vi "Measurement UI.vi"() -> ()   [LabVIEW 2021, in "Eff And Load Reg_Channel Ganging_UI.lvlib"]
uses:
  Eff And Load Reg_Channel Ganging_UI.lvlib
panel:
  in  "MeasGraphs":T1(tab)
  out "EfficiencyGraph":T2(graph)
  out "LoadRegulationGraph(V/A)":T3(graph)
  out "LoadRegulationGraph(%)":T3(graph)
  out "Load voltage deviation":dbl[](array[numeric])
  out "Ganged load voltages":dbl[](array[numeric])
  in  "Load current pole-zero ratio":dbl=0.3
  in  "Load current compensation frequency":dbl=180000.0
  in  "Load current gain bandwidth":dbl=14000.0
  in  "Source voltage pole-zero ratio":dbl=2.0
  in  "Source voltage compensation frequency":dbl=3530.0
  in  "Source voltage gain bandwidth":dbl=2000.0
  in  "Load resource names":string[](array[string])
  in  "Source resource names":string[](array[string])
  out "Load sweep points":i32
  out "Source sweep points":i32
  out "Voltage values":dbl[](array[numeric])
  out "Efficiency":dbl[](array[numeric])
  out "Ganged load currents":dbl[](array[numeric])
  in  "Mode of operation":T4(ring)
  in  "ModeOfConfiguration":T5(tab)
  in  "DEVICE POWER":bool=TRUE
  out "Status":string
  in  "Load config power on":string="Load Config"
  in  "POWERON/OFFLOADResourceNames":refnum<k15>[](array[refnum]) caption="RESOURCE NAMES"
  in  "Source config power on":string="Source Config"
  in  "POWERON/ OFFSOURCEResourceNames":refnum<k15>[](array[refnum]) caption="RESOURCE NAMES\n(Single/Master & Slave)"
  in  "Power on source sense":i32(ring)=1009 caption="SENSE" items=["Local"=1008, "Remote"=1009]
  in  "Power on/off Source voltage/current limit range":dbl=15.0 caption="CURRENT LIMIT" format="%#_6pA"
  in  "Power on/off Source voltage/current level":dbl=6.0 caption="VOLTAGE LEVEL" format="%#_6pV"
  in  "Power on source system configuration":enum32{"Series", "Parallel"}(ring)=enum."Parallel" caption="SYSTEM CONFIG"
  in  "Power ON output function":i32(ring)=1006 caption="OUTPUT FUNCTION" items=["DC Voltage"=1006, "DC Current"=1007]
  in  "MeasConfigurations":T6(tab)=enum."Source Config"
  in  "Measurement timeout":dbl=10.0 caption="MEASUREMENT TIME-OUT" format="%.3ps"
  in  "Nominal output voltage":dbl=1.0 caption="NOMINAL OUTPUT VOLTAGE" format="%.3fV"
  in  "Source delay":dbl=0.005 caption="SOURCE DELAY" format="%.3ps"
  in  "DUT setup time":dbl=1.0 caption="DUT SETUP TIME" format="%.3ps"
  in  "Aperture time":dbl=0.005 caption="APERTURE TIME" format="%.3ps"
  in  "PPSSResourceNames":refnum<k15>[](array[refnum]) caption="RESOURCE NAMES"
  in  "Source stop voltage":dbl=14.0 caption="VOLTAGE STOP LEVEL" format="%#_6pV"
  in  "Source transient response":i32(ring)=1038 caption="TRANSIENT RESPONSE" items=["Slow"=1041, "Normal"=1038, "Fast"=1039, "Custom"=1042]
  in  "Power ON/Source sense":i32(ring)=1009 caption="SENSE" items=["Local"=1008, "Remote"=1009]
  in  "Source voltage level range":dbl=20.0 caption="VOLTAGE LEVEL RANGE" format="%#_6pV"
  in  "Power ON V/I Source start level":dbl=6.0 caption="VOLTAGE START LEVEL" format="%#_6pV"
  in  "Source current limit high":dbl=25.0 caption="CURRENT LIMIT/LIMIT HIGH" format="%#_6pA"
  in  "Power ON/Source current/voltage limit range":dbl=25.0 caption="CURRENT LIMIT RANGE" format="%#_6pA"
  in  "Source limit symmetry":enum32{"Symmetric", "Asymmetric"}(ring)=enum."Asymmetric" caption="LIMIT SYMMETRY"
  in  "Source current limit low":dbl=-0.6 caption="CURRENT LIMIT LOW" format="%#_6pA"
  in  "Power ON/Source system configuration":enum32{"Series", "Parallel"}(ring)=enum."Parallel" caption="SYSTEM CONFIG"
  in  "Source compliance":string="Compliance"
  in  "Source sourceadapt":string="SourceAdapt"
  in  "Source voltage sweep points":i32=4 caption="NO. OF POINTS"
  in  "Source Custom Transient Response":bool
  in  "Load current sweep points/points per decade":i32=10 caption="PTS/PTS PER DECADE"
  in  "Load sweep type":string(combo)="Logarithmic" caption="SWEEP TYPE"
  in  "Load stop current":dbl=50.0 caption="CURRENT STOP LEVEL" format="%#_6pA"
  in  "Load sourceadapt":string="SourceAdapt"
  in  "Load compliance":string="Compliance"
  in  "Load system configuration":enum32{"Series", "Parallel"}(ring)=enum."Parallel" caption="SYSTEM CONFIG"
  in  "Load voltage limit low":dbl caption="VOLTAGE  LIMIT LOW" format="%#_6pV"
  in  "Load limit symmetry":enum32{"Symmetric", "Asymmetric"}(ring) caption="LIMIT SYMMETRY"
  in  "Load voltage limit range":dbl=6.0 caption="VOLTAGE LIMIT RANGE" format="%#_6pV"
  in  "Load voltage limit high":dbl=inf caption="VOLTAGE LIMIT/LIMIT HIGH" format="%#_6p"
  in  "Load start current":dbl=2.0 caption="CURRENT START LEVEL" format="%#_6pA"
  in  "Load current level range":dbl=80.0 caption="CURRENT LEVEL RANGE" format="%#_6pA"
  in  "Load sense":i32(ring)=1009 caption="SENSE" items=["Local"=1008, "Remote"=1009]
  in  "Load transient response":i32(ring)=1038 caption="TRANSIENT RESPONSE" items=["Slow"=1041, "Normal"=1038, "Fast"=1039, "Custom"=1042]
  in  "ELoad resource names":refnum<k15>[](array[refnum]) caption="RESOURCE NAMES"
  in  "Load Custom Transient Response":bool
  in  "Load device voltage/current rating":dbl=50.0 caption="DEVICE CURRENT RATING" format="%#_6pA"
  out "Eload status":string
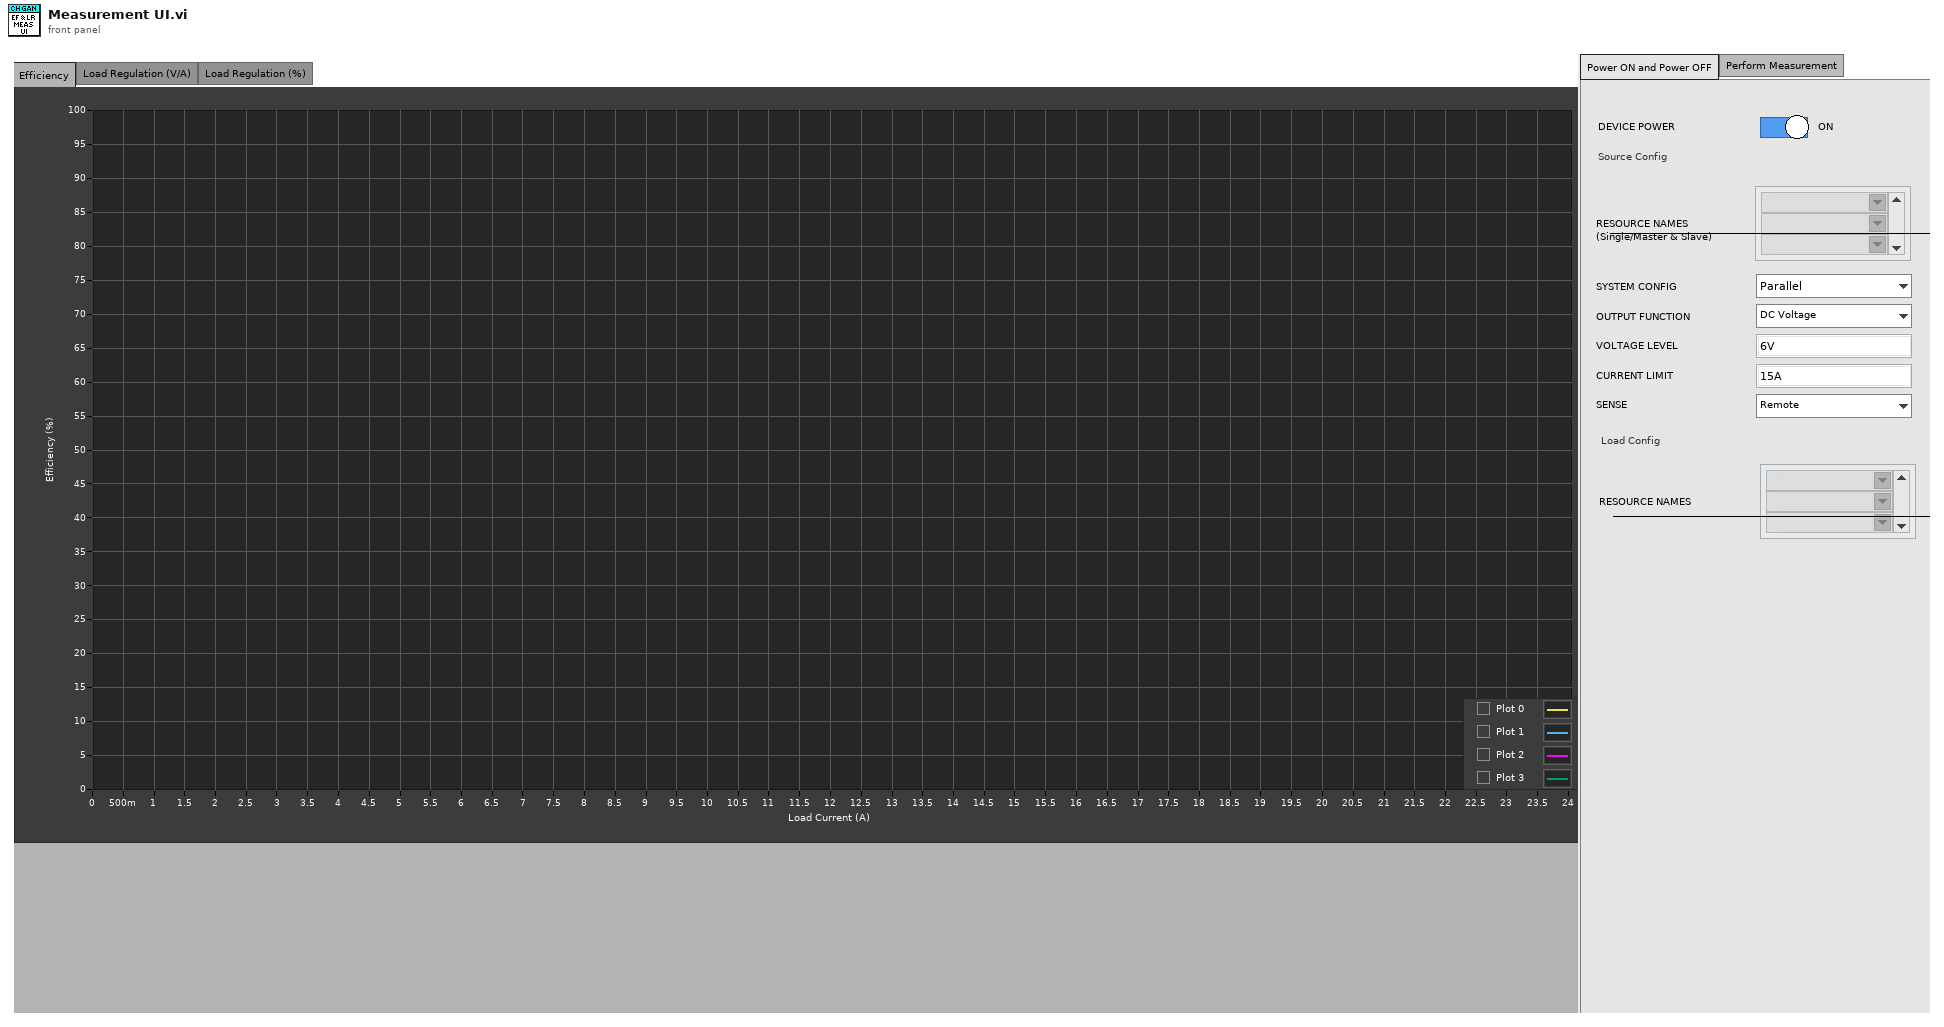
[diagram p1: front panel]
types:
  T1 = enum32{"Efficiency", "Load Regulation (V/A)", "Load Regulation (%)", "Hidden Controls"}
  T2 = cluster{"Ganged load currents":dbl[], "Efficiency":dbl[]}[]
  T3 = cluster{"Load currents":dbl[], "Efficiency":dbl[]}[]
  T4 = enum32{"Power on the DUT", "Perform measurement", "Power off the DUT"}
  T5 = enum32{"Power ON and Power OFF", "Perform Measurement"}
  T6 = enum32{"Measurement Config", "Source Config", "Load Config"}
  T7 = typedef "SourceAdapt Parameters.ctl" = cluster{"Voltage gain bandwidth":dbl, "Voltage compensation frequency":dbl, "Voltage pole-zero ratio":dbl, "Current gain bandwidth":dbl, "Current compensation frequency":dbl, "Current pole-zero ratio":dbl}
  T8 = cluster{"Ganged load currents":dbl[], "Efficiency":dbl[]}
  T9 = cluster{"Ganged load currents":dbl[], "Ganged load voltages":dbl[]}
  T10 = cluster{"Ganged load currents":dbl[], "Load voltage deviation":dbl[]}
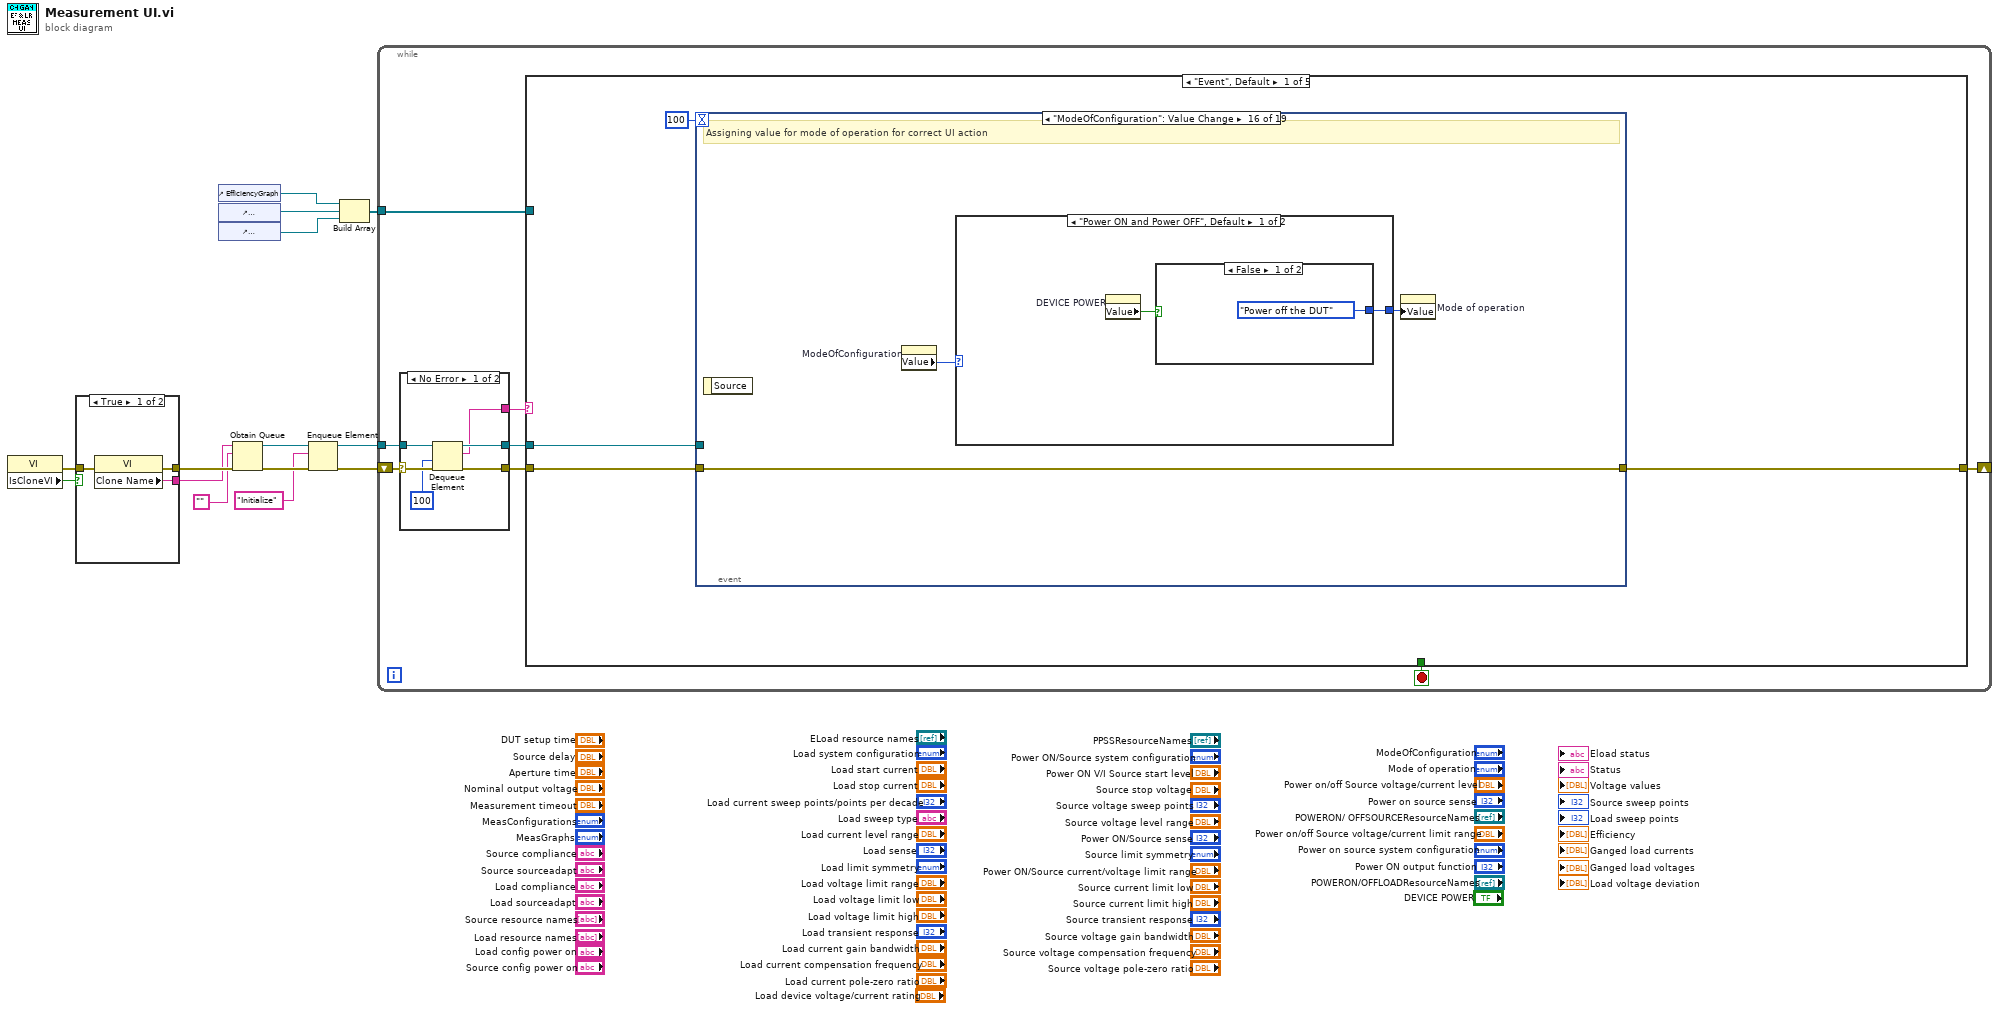
[diagram p0: block diagram]
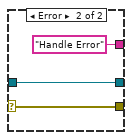
[diagram p2: hidden frame]
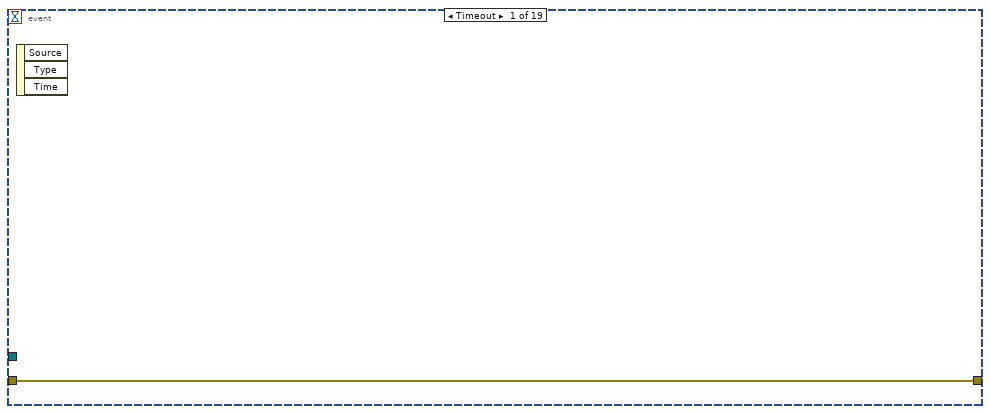
[diagram p3: hidden frame]
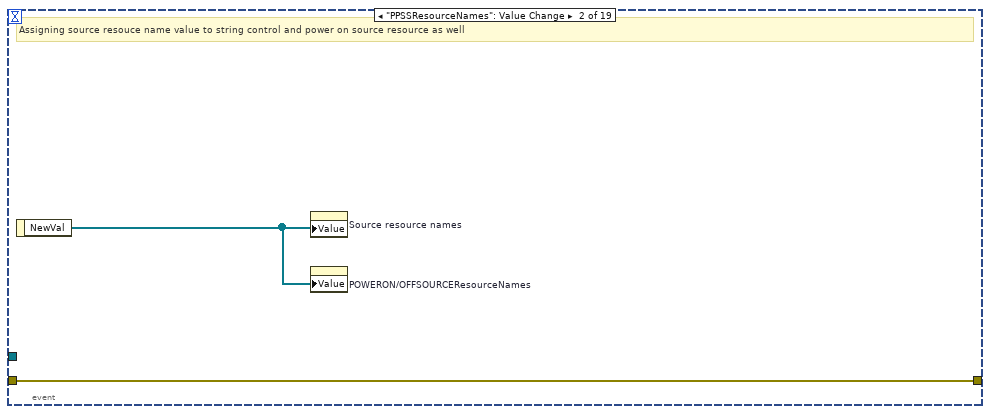
[diagram p4: hidden frame]
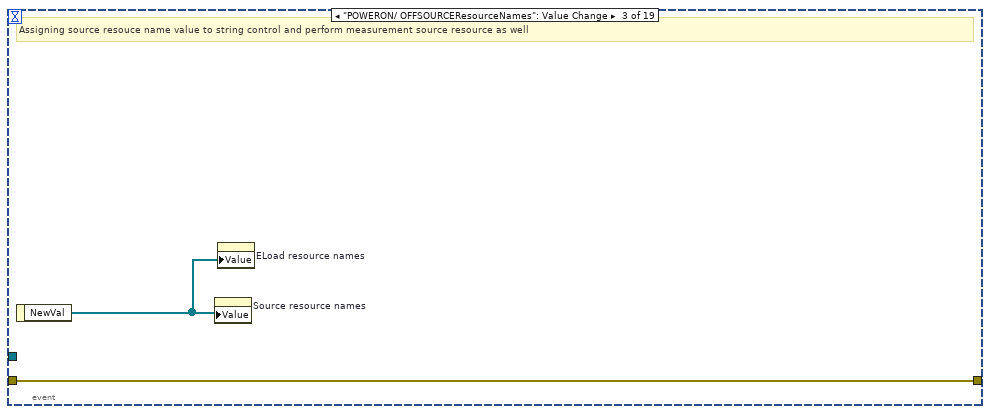
[diagram p5: hidden frame]
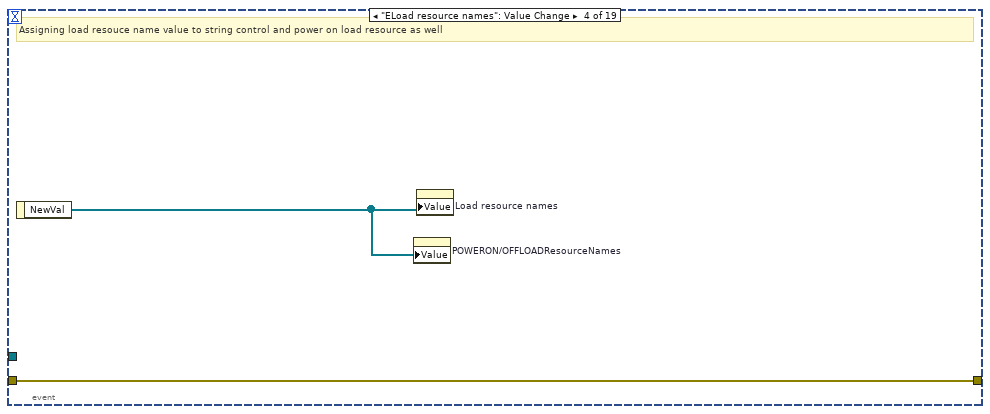
[diagram p6: hidden frame]
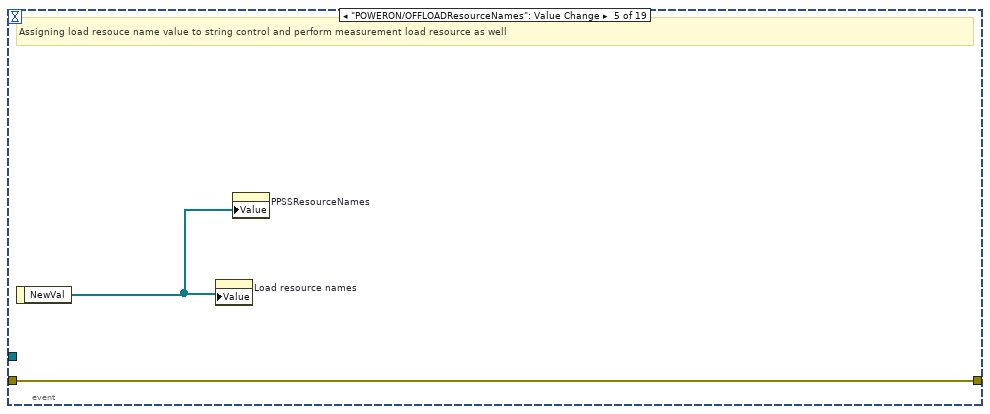
[diagram p7: hidden frame]
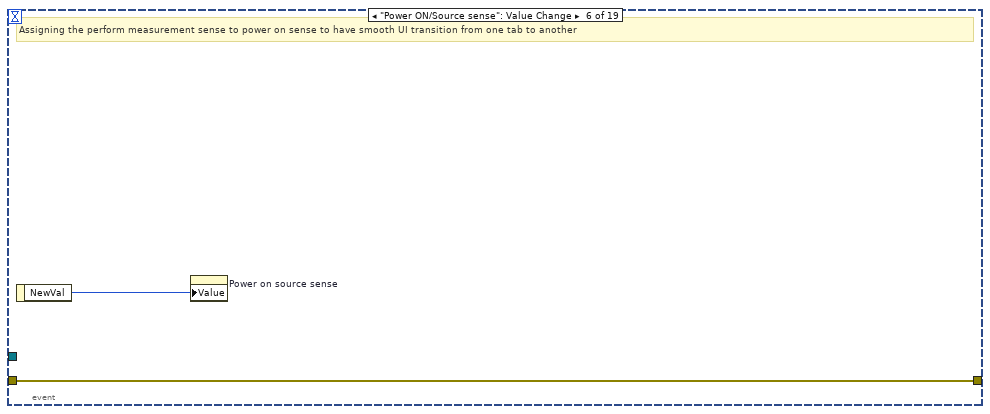
[diagram p8: hidden frame]
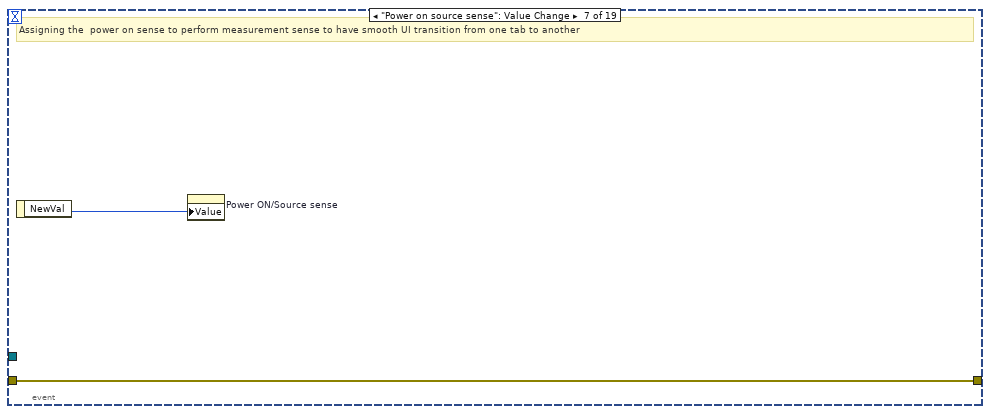
[diagram p9: hidden frame]
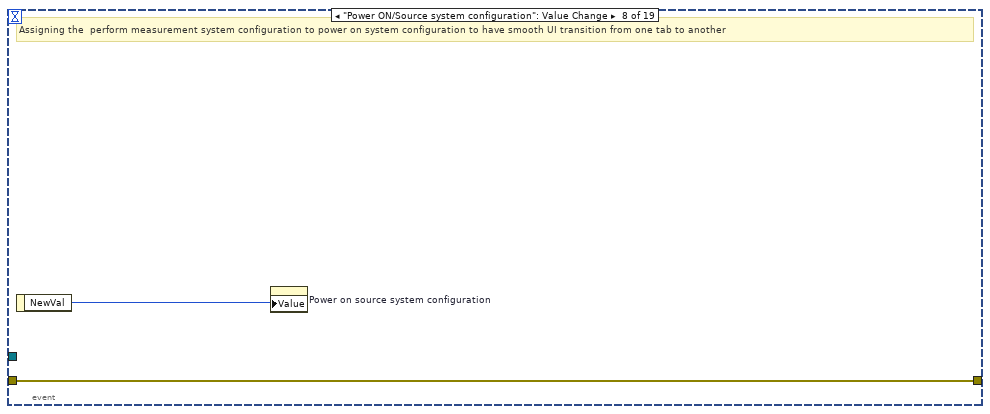
[diagram p10: hidden frame]
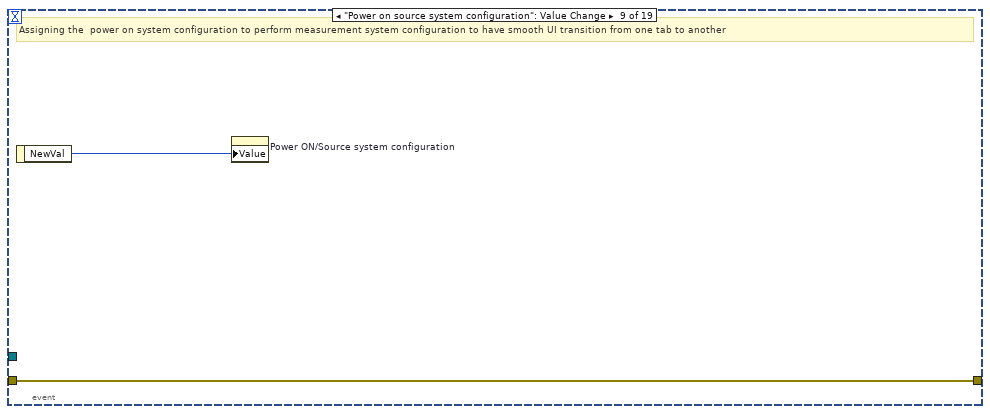
[diagram p11: hidden frame]
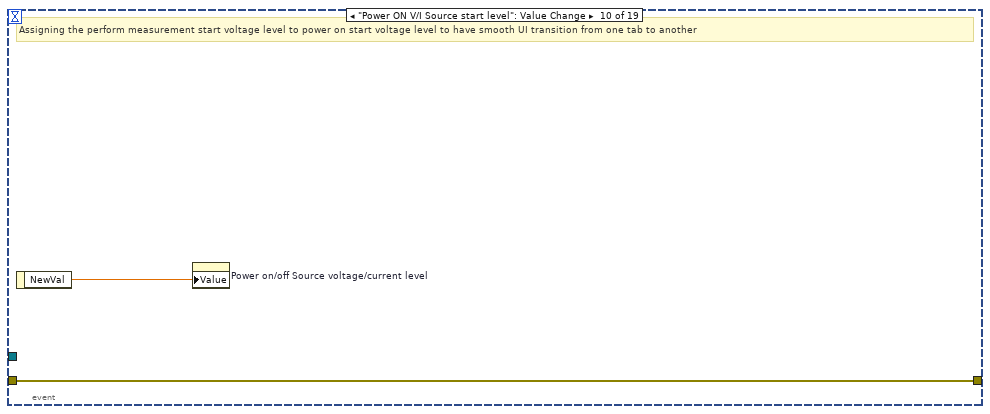
[diagram p12: hidden frame]
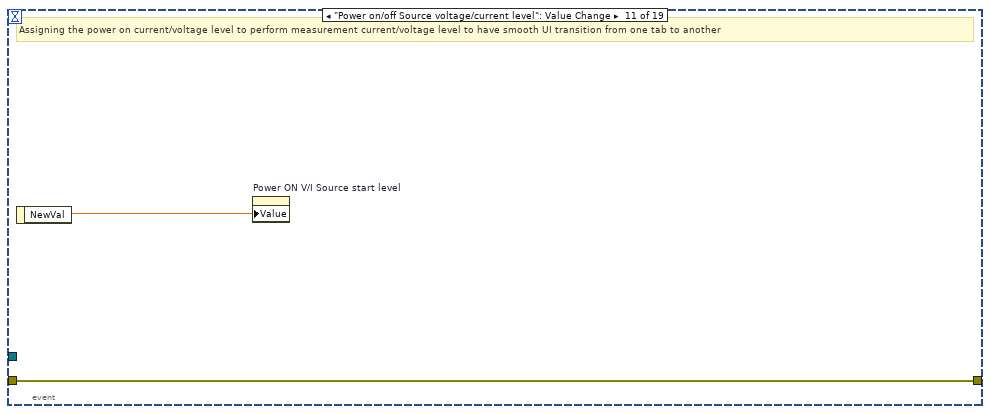
[diagram p13: hidden frame]
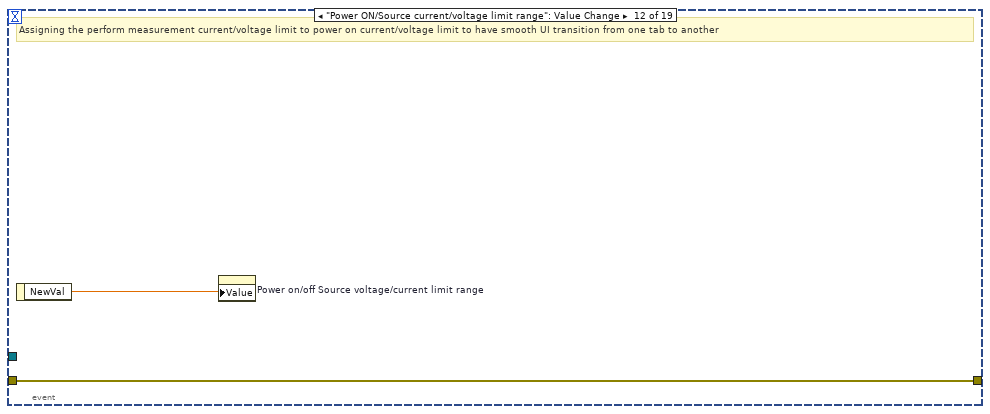
[diagram p14: hidden frame]
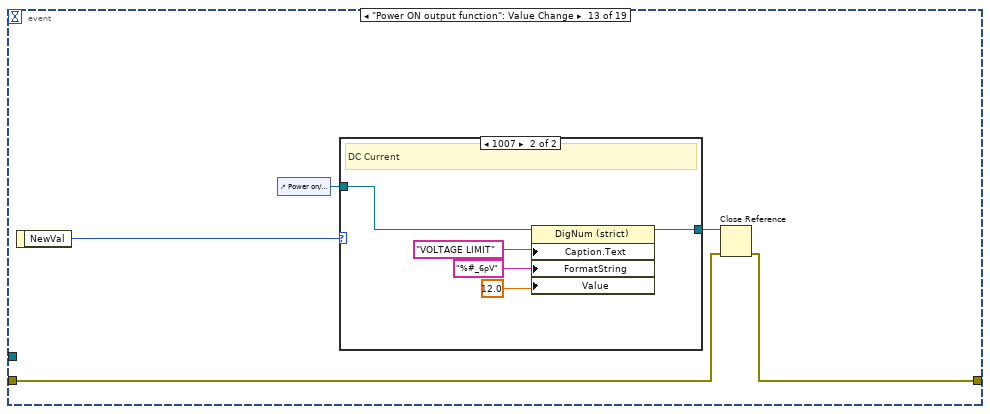
[diagram p15: hidden frame]
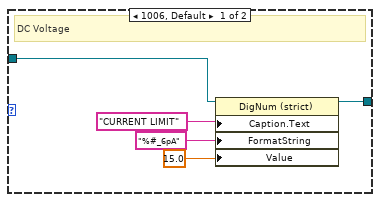
[diagram p16: hidden frame]
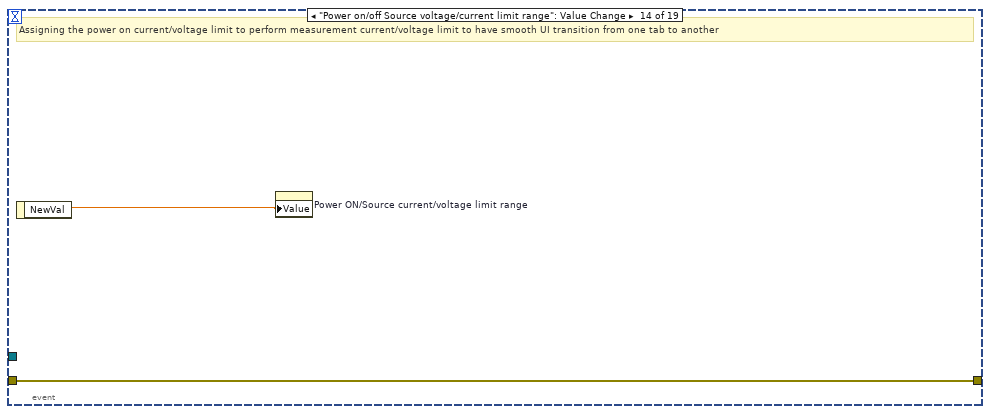
[diagram p17: hidden frame]
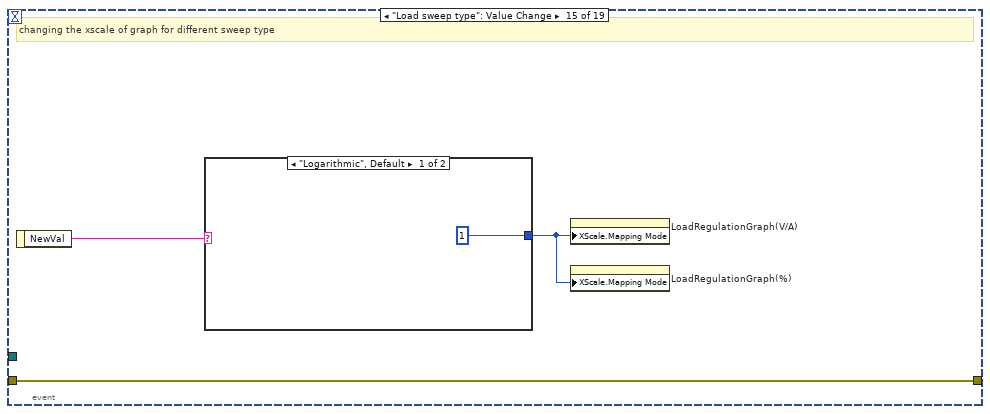
[diagram p18: hidden frame]
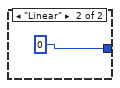
[diagram p19: hidden frame]
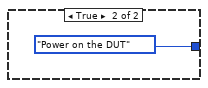
[diagram p20: hidden frame]
diagram:
  n1 = property class="VI"() -> (error out=w5:errorcluster, "IsCloneVI"=w6:bool)  [unwired: 2 in, 1 out]
  n2 = case shown="True" w6 {
    tunnel: [w17 w20] -> w14
    tunnel: [w16 w19] -> w13
    tunnel: w5 -> [w15 w18]
    frame True {
      n3 = property class="VI"(error in=w15) -> (error out=w17:errorcluster, "Clone Name"=w16:string)  [unwired: 1 in, 1 out]
    }
    frame False {
      n4 = property class="VI"(error in=w18) -> (error out=w20:errorcluster, "Name"=w19:string)  [unwired: 1 in, 1 out]
    }
  }
  n5 = control-ref of="EfficiencyGraph"() -> (w2:refnum<vi>)
  n6 = control-ref of="LoadRegulationGraph(V/A)"() -> (w3:refnum<vi>)
  n7 = control-ref of="LoadRegulationGraph(%)"() -> (w4:refnum<vi>)
  n8 = Obtain Queue(name (unnamed)=w13, element data type="", error in (no error)=w14) -> (queue out=w10:refnum<queue>, error out=w12:errorcluster)  [unwired: 2 in, 1 out]
  n9 = Enqueue Element(queue=w10, element="Initialize", error in (no error)=w12) -> (queue out=w9:refnum<queue>, error out=w11:errorcluster)  [unwired: 1 in, 1 out]
  n10 = Build Array(w2, w3, w4) -> (w1:refnum<vi>[])
  n11 = while {
    shift-right: [w23] -> _
    shift-left: w11 -> [w28]
    tunnel: w9 -> [w26]
    tunnel: w1 -> [w21]
    stop <- w22 stop-if-true
    n12 = case shown="No Error" w28 {
      selector: w28 -> [w34 w37]
      tunnel: [w33 w37] -> w27
      tunnel: w26 -> [w32 w36]
      tunnel: [w31 w36] -> w25
      tunnel: [w30 "Handle Error"] -> w24
      frame No Error {
        n13 = Dequeue Element(queue=w32, timeout in ms (-1)=100, error in (no error)=w34) -> (queue out=w31:refnum<queue>, element=w30:string, error out=w33:errorcluster)  [unwired: 1 out]
      }
      frame Error {
      }
    }
    n14 = case shown="\"Event\", Default" w24 {
      tunnel: w27 -> [w40 w110 w125 w182 w183]
      tunnel: w25 -> [w38 _ _ w180 _]
      tunnel: [w41 w110 w125 w177 w183] -> w23
      tunnel: [_ _ _ TRUE _] -> w22
      tunnel: w21 -> [_ _ w113 _ _]
      frame "Event", Default {
        n15 = event shown="[15] \"ModeOfConfiguration\": Value Change" {
          selector: _ -> [_ _ _ _ _ _ _ _ _ _ _ _ _ _ _ _ _ _ _]
          dyn-events: _ -> [_ _ _ _ _ _ _ _ _ _ _ _ _ _ _ _ _ _ _]
          timeout: 100 -> [_ _ _ _ _ _ _ _ _ _ _ _ _ _ _ _ _ _ _]
          tunnel: [w42 w44 w46 w48 w49 w51 w53 w55 w57 w59 w61 w63 w65 w81 w82 w87 w98 w103 w107] -> w41
          tunnel: w40 -> [w42 w44 w46 w48 w49 w51 w53 w55 w57 w59 w61 w63 w66 w81 w82 w87 w98 w103 w108]
          tunnel: w38 -> [_ _ _ _ _ _ _ _ _ _ _ _ _ _ _ _ _ _ w106]
          event Timeout {
            n16 = event-data() -> ()  [unwired: 1 in, 3 out]
          }
          event "PPSSResourceNames": Value Change {
            # "Assigning source resouce name value to string control and power on source resource as well"
            n17 = event-data() -> ("NewVal"=w43:refnum<k15>[])  [unwired: 1 in]
            n18 = property on="Source resource names" class="Arr (strict)"("Value"=w43) -> ()  [unwired: 2 in, 2 out]
            n19 = property on="POWERON/OFFSOURCEResourceNames" class="Arr (strict)"("Value"=w43) -> ()  [unwired: 2 in, 2 out]
          }
          event "POWERON/ OFFSOURCEResourceNames": Value Change {
            # "Assigning source resouce name value to string control and perform measurement source resource as well"
            n20 = event-data() -> ("NewVal"=w45:refnum<k15>[])  [unwired: 1 in]
            n21 = property on="Source resource names" class="Arr (strict)"("Value"=w45) -> ()  [unwired: 2 in, 2 out]
            n22 = property on="ELoad resource names" class="Arr (strict)"("Value"=w45) -> ()  [unwired: 2 in, 2 out]
          }
          event "ELoad resource names": Value Change {
            # "Assigning load resouce name value to string control and power on load resource as well"
            n23 = event-data() -> ("NewVal"=w47:refnum<k15>[])  [unwired: 1 in]
            n24 = property on="POWERON/OFFLOADResourceNames" class="Arr (strict)"("Value"=w47) -> ()  [unwired: 2 in, 2 out]
            n25 = property on="Load resource names" class="Arr (strict)"("Value"=w47) -> ()  [unwired: 2 in, 2 out]
          }
          event "POWERON/OFFLOADResourceNames": Value Change {
            # "Assigning load resouce name value to string control and perform measurement load resource as well"
            n26 = event-data() -> ("NewVal"=w50:refnum<k15>[])  [unwired: 1 in]
            n27 = property on="Load resource names" class="Arr (strict)"("Value"=w50) -> ()  [unwired: 2 in, 2 out]
            n28 = property on="PPSSResourceNames" class="Arr (strict)"("Value"=w50) -> ()  [unwired: 2 in, 2 out]
          }
          event "Power ON/Source sense": Value Change {
            # "Assigning the perform measurement sense to power on sense to have smooth UI transition from one tab to another"
            n29 = event-data() -> ("NewVal"=w52:i32)  [unwired: 1 in]
            n30 = property on="Power on source sense" class="Ring (strict)"("Value"=w52) -> ()  [unwired: 2 in, 2 out]
          }
          event "Power on source sense": Value Change {
            # "Assigning the  power on sense to perform measurement sense to have smooth UI transition from one tab to another"
            n31 = event-data() -> ("NewVal"=w54:i32)  [unwired: 1 in]
            n32 = property on="Power ON/Source sense" class="Ring (strict)"("Value"=w54) -> ()  [unwired: 2 in, 2 out]
          }
          event "Power ON/Source system configuration": Value Change {
            # "Assigning the  perform measurement system configuration to power on system configuration to have smooth UI transition from one tab to another"
            n33 = event-data() -> ("NewVal"=w56:enum32{"Series", "Parallel"})  [unwired: 1 in]
            n34 = property on="Power on source system configuration" class="Enum (strict)"("Value"=w56) -> ()  [unwired: 2 in, 2 out]
          }
          event "Power on source system configuration": Value Change {
            # "Assigning the  power on system configuration to perform measurement system configuration to have smooth UI transition from one tab to another"
            n35 = event-data() -> ("NewVal"=w58:enum32{"Series", "Parallel"})  [unwired: 1 in]
            n36 = property on="Power ON/Source system configuration" class="Enum (strict)"("Value"=w58) -> ()  [unwired: 2 in, 2 out]
          }
          event "Power ON V/I Source start level": Value Change {
            # "Assigning the perform measurement start voltage level to power on start voltage level to have smooth UI transition from one tab to another"
            n37 = event-data() -> ("NewVal"=w60:dbl)  [unwired: 1 in]
            n38 = property on="Power on/off Source voltage/current level" class="DigNum (strict)"("Value"=w60) -> ()  [unwired: 2 in, 2 out]
          }
          event "Power on/off Source voltage/current level": Value Change {
            # "Assigning the power on current/voltage level to perform measurement current/voltage level to have smooth UI transition from one tab to another"
            n39 = event-data() -> ("NewVal"=w62:dbl)  [unwired: 1 in]
            n40 = property on="Power ON V/I Source start level" class="DigNum (strict)"("Value"=w62) -> ()  [unwired: 2 in, 2 out]
          }
          event "Power ON/Source current/voltage limit range": Value Change {
            # "Assigning the perform measurement current/voltage limit to power on current/voltage limit to have smooth UI transition from one tab to another"
            n41 = event-data() -> ("NewVal"=w64:dbl)  [unwired: 1 in]
            n42 = property on="Power on/off Source voltage/current limit range" class="DigNum (strict)"("Value"=w64) -> ()  [unwired: 2 in, 2 out]
          }
          event "Power ON output function": Value Change {
            n43 = event-data() -> ("NewVal"=w69:i32)  [unwired: 1 in]
            n44 = control-ref of="Power on/off Source voltage/current limit range"() -> (w68:refnum<vi>)
            n45 = case shown="1007" w69 {
              tunnel: w68 -> [w73 w79]
              tunnel: [w74 w78] -> w67
              frame 1006, Default {
                # "DC Voltage"
                n46 = property class="DigNum (strict)"(reference=w73, "Caption.Text"="CURRENT LIMIT", "FormatString"="%#_6pA" ("Format String"), "Value"=15.0) -> (reference out=w74:refnum<vi>)  [unwired: 1 in, 1 out]
              }
              frame 1007 {
                # "DC Current"
                n47 = property class="DigNum (strict)"(reference=w79, "Caption.Text"="VOLTAGE LIMIT", "FormatString"="%#_6pV" ("Format String"), "Value"=12.0) -> (reference out=w78:refnum<vi>)  [unwired: 1 in, 1 out]
              }
            }
            n48 = Close Reference(reference=w67, error in (no error)=w66) -> (error out=w65:errorcluster)
          }
          event "Power on/off Source voltage/current limit range": Value Change {
            # "Assigning the power on current/voltage limit to perform measurement current/voltage limit to have smooth UI transition from one tab to another"
            n49 = event-data() -> ("NewVal"=w80:dbl)  [unwired: 1 in]
            n50 = property on="Power ON/Source current/voltage limit range" class="DigNum (strict)"("Value"=w80) -> ()  [unwired: 2 in, 2 out]
          }
          event "Load sweep type": Value Change {
            # "changing the xscale of graph for different sweep type"
            n51 = event-data() -> ("NewVal"=w84:string)  [unwired: 1 in]
            n52 = case shown="\"Logarithmic\", Default" w84 {
              tunnel: [u8 1 ("X Scale.Mapping Mode") u8 0 ("X Scale.Mapping Mode")] -> w83
              frame "Logarithmic", Default {
              }
              frame "Linear" {
              }
            }
            n53 = property on="LoadRegulationGraph(V/A)" class="XYGraph (strict)"("XScale.Mapping Mode"=w83) -> ()  [unwired: 2 in, 2 out]
            n54 = property on="LoadRegulationGraph(%)" class="XYGraph (strict)"("XScale.Mapping Mode"=w83) -> ()  [unwired: 2 in, 2 out]
          }
          event "ModeOfConfiguration": Value Change {
            # "Assigning value for mode of operation for correct UI action"
            n55 = event-data() -> ()  [unwired: 1 in, 1 out]
            n56 = property on="ModeOfConfiguration" class="TabCtl (strict)"() -> ("Value"=w89:T5)  [unwired: 2 in, 2 out]
            n57 = case shown="\"Power ON and Power OFF\", Default" w89 {
              tunnel: [w91 T4."Perform measurement" ("Mode of operation")] -> w88
              frame "Power ON and Power OFF", Default {
                n58 = property on="DEVICE POWER" class="Bool (strict)"() -> ("Value"=w90:bool)  [unwired: 2 in, 2 out]
                n59 = case shown="False" w90 {
                  tunnel: [T4."Power off the DUT" ("Mode of operation") T4."Power on the DUT" ("Mode of operation")] -> w91
                  frame False {
                  }
                  frame True {
                  }
                }
              }
              frame "Perform Measurement" {
              }
            }
            n60 = property on="Mode of operation" class="Enum (strict)"("Value"=w88) -> ()  [unwired: 2 in, 2 out]
          }
          event "Source Custom Transient Response": Value Change {
            # "transient paramter assigned"
            n61 = event-data() -> ()  [unwired: 1 in, 6 out]
            n62 = call "Custom Transient Response for Sweep & Single Point.vi"() -> ("SourceAdapt Parameters"=w99:T7)  [unwired: 11 in]
            n63 = Unbundle By Name(w99) -> ("Voltage gain bandwidth"=w96:dbl, "Voltage compensation frequency"=w97:dbl, "Voltage pole-zero ratio"=w95:dbl)
            n64 = property on="Source voltage gain bandwidth" class="DigNum (strict)"("Value"=w96) -> ()  [unwired: 2 in, 2 out]
            n65 = property on="Source voltage compensation frequency" class="DigNum (strict)"("Value"=w97) -> ()  [unwired: 2 in, 2 out]
            n66 = property on="Source voltage pole-zero ratio" class="DigNum (strict)"("Value"=w95) -> ()  [unwired: 2 in, 2 out]
          }
          event "Load Custom Transient Response": Value Change {
            # "transient paramter assigned"
            n67 = event-data() -> ()  [unwired: 1 in, 6 out]
            n68 = call "Custom Transient Response for Sweep & Single Point.vi"() -> ("SourceAdapt Parameters"=w104:T7)  [unwired: 11 in]
            n69 = Unbundle By Name(w104) -> ("Current gain bandwidth"=w100:dbl, "Current compensation frequency"=w102:dbl, "Current pole-zero ratio"=w101:dbl)
            n70 = property on="Load current gain bandwidth" class="DigNum (strict)"("Value"=w100) -> ()  [unwired: 2 in, 2 out]
            n71 = property on="Load current compensation frequency" class="DigNum (strict)"("Value"=w102) -> ()  [unwired: 2 in, 2 out]
            n72 = property on="Load current pole-zero ratio" class="DigNum (strict)"("Value"=w101) -> ()  [unwired: 2 in, 2 out]
          }
          event Panel Close? {
            n73 = event-data() -> ()  [unwired: 1 in, 4 out]
            n74 = Enqueue Element(queue=w106, element="Exit", error in (no error)=w108) -> (error out=w107:errorcluster)  [unwired: 1 in, 2 out]
            n75 = event-data("Discard?"=TRUE) -> ()  [unwired: 1 in, 1 out]
          }
        }
      }
      frame "Initialize" {
      }
      frame "Post UI Update" {
        w120 = u32[] [15787074, 5682409, 15535092, 40563, 13983232, 35009, 15113984, 13400487, 15993633, 10221451, 8148942, 15869817, 32914, 10196480, 6271923, 16355671]  # Plot colors
        # "This case will be triggered, after framework updates the User interface with result values."
        n76 = local read "Source sweep points"() -> (w118:i32)
        n77 = local read "Voltage values"() -> (w119:dbl[])
        n78 = for {
          tunnel: w120 -> [w130]
          tunnel: w113 -> [w129] mode=indexing
          tunnel: w119 -> [w128]
          tunnel: w118 -> [w127]
          tunnel: [w126] -> w112
          n79 = for {
            tunnel: w128 -> [w143] mode=indexing
            tunnel: [w143] -> w126 mode=indexing
            tunnel: w129 -> [w136]
            tunnel: w127 -> [w133]
            tunnel: w130 -> [w139] mode=indexing
            i -> [w137]
            n80 = Greater?(x=w137, y=3) -> (0:w141:bool)
            n81 = To Unsigned Long Integer(number=w137) -> (unsigned 32bit integer=w140:u32)
            n82 = Increment(x=w137) -> (x+1=w135:i32)
            n83 = Format Value(format string="%.3f", value (0)=w143) -> (output string=w146:string)  [unwired: 1 out]
            n84 = case shown="False" w141 {
              tunnel: w136 -> [w152 w158]
              tunnel: w135 -> [w151 _]
              tunnel: [w150 w157] -> w134
              tunnel: w133 -> [w148 w153]
              tunnel: [w149 w156] -> w132
              frame False {
                # "Color selector for less than 3ch"
                n85 = property on="Property Node" class="XYGraph (strict)"(reference=w152, "LegScrollVis"=FALSE ("Legend:Scrollbar Visible"), "LegNumRows"=w151, "LegPlotMin"=w148) -> (reference out=w150:refnum<vi>, error out=w149:errorcluster)  [unwired: 1 in]
              }
              frame True {
                # "Color selector for more than 3ch"
                n86 = property on="Property Node" class="XYGraph (strict)"(reference=w158, "LegScrollVis"=TRUE ("Legend:Scrollbar Visible"), "LegNumRows"=u32 4 ("Legend:Number of Rows"), "LegPlotMin"=w153) -> (reference out=w157:refnum<vi>, error out=w156:errorcluster)  [unwired: 1 in]
              }
            }
            n87 = Concatenate Strings(" Vin = " ("string"), w146) -> (w131:string)
            n88 = property on="Property Node" class="XYGraph (strict)"(reference=w134, error in=w132, "Active Plot"=w140, "Plot.Point Style"=u8 5, "Plot.Plot Color"=w139, "Plot.Fill/Pt. Color"=w139, "Plot.Plot Name"=w131) -> ()  [unwired: 2 out]
          }
        }
        n89 = local read "Load voltage deviation"() -> (w116:dbl[])
        n90 = local read "Ganged load currents"() -> (w124:dbl[])
        n91 = local read "Ganged load voltages"() -> (w117:dbl[])
        n92 = local read "Load sweep points"() -> (w121:i32)
        n93 = Array Size(array=w112) -> (size(s)=w111:i32)
        n94 = local read "Efficiency"() -> (w123:dbl[])
        n95 = for {
          N: w111 -> [_]
          tunnel: [w175] -> w122 mode=indexing
          shift-right: [w174] -> _
          shift-left: w124 -> [w172]
          shift-right: [w170] -> _
          shift-left: w123 -> [w171]
          tunnel: w121 -> [w169]
          shift-right: [w166] -> _
          shift-left: w117 -> [w168]
          shift-right: [w163] -> _
          shift-left: w116 -> [w167]
          tunnel: [w162] -> w114 mode=indexing
          tunnel: [w161] -> w115 mode=indexing
          w160 = 0 ("index")
          n96 = Delete From Array(array=w172, length=w169, index=w160) -> (deleted portion=w164:dbl[], array with subset deleted=w174:dbl[])
          n97 = Delete From Array(array=w171, length=w169, index=w160) -> (deleted portion=w173:dbl[], array with subset deleted=w170:dbl[])
          n98 = Delete From Array(array=w168, length=w169, index=w160) -> (deleted portion=w165:dbl[], array with subset deleted=w166:dbl[])
          n99 = Delete From Array(array=w167, length=w169, index=w160) -> (deleted portion=w159:dbl[], array with subset deleted=w163:dbl[])
          n100 = Bundle("Ganged load currents"=w164, "Efficiency"=w173) -> (w175:T8)  [unwired: 1 in]
          n101 = Bundle("Ganged load currents"=w164, "Ganged load voltages"=w165) -> (w161:T9)  [unwired: 1 in]
          n102 = Bundle("Ganged load currents"=w164, "Load voltage deviation"=w159) -> (w162:T10)  [unwired: 1 in]
        }
        "EfficiencyGraph" <- w122
        "LoadRegulationGraph(V/A)" <- w115
        "LoadRegulationGraph(%)" <- w114
      }
      frame "Exit" {
        # "This case is triggered to close the User Interface from framework"
        n103 = Flush Queue(queue=w180, error in (no error)=w182) -> (queue out=w179:refnum<queue>, error out=w178:errorcluster)  [unwired: 1 out]
        n104 = Release Queue(queue=w179, force destroy? (F)=TRUE, error in (no error)=w178) -> (error out=w177:errorcluster)  [unwired: 2 out]
      }
      frame "Handle Error" {
      }
    }
  }
